vi "Read Config InI.vi"(0 "名称或相对路径":string="UserDefine.ini", 5 "error in (no error)":errorcluster caption="错误输入（无错误）") -> (14 "ParamSet":string[](array[string]), 15 "Other Params":string[](array[string]), 17 "In Stack":string[](array[string]), 18 "Out Stack":string[](array[string]), 19 "error out":errorcluster caption="错误输出")   [LabVIEW 2017]
uses:
  Global System.vi
  <vilib>/Utility/config.llb/NI_LVConfig.lvlib
panel:
  out "添加的路径":path
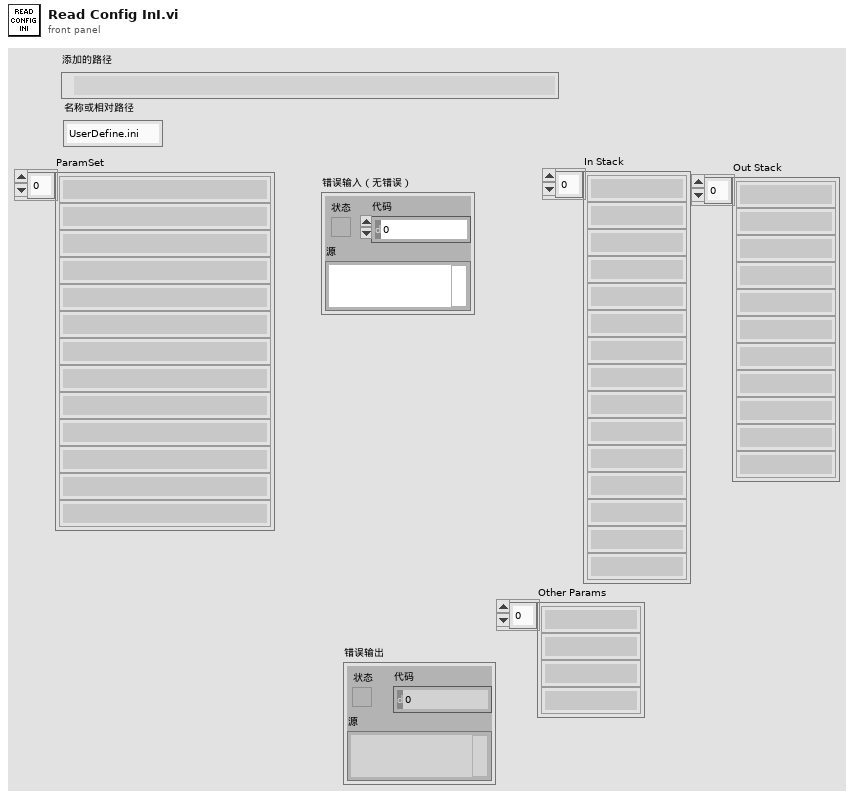
[diagram p1: front panel]
types:
  T1 = typedef "NI_LVConfig.lvlib/Config Data RefNum.ctl" = refnum<k1>
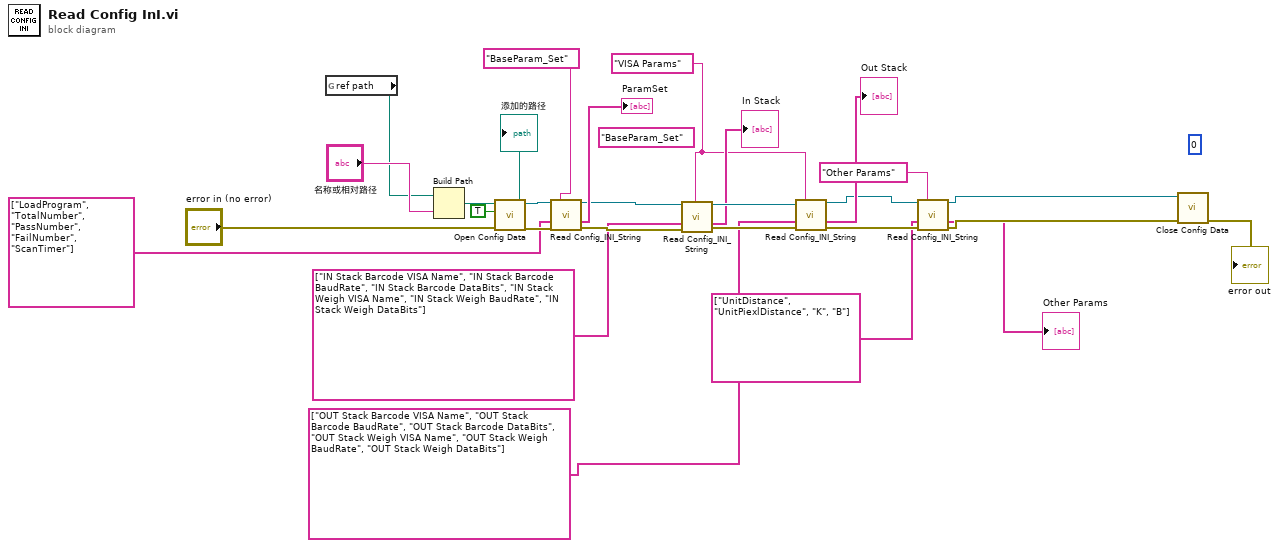
[diagram p0: block diagram]
diagram:
  w8 = "VISA Params" ("section")
  (unwired) "BaseParam_Set" ("section")
  (unwired) 0 ("索引")
  n1 = global read "Global System.vi" "ref path"() -> (w21:path)
  n2 = Build Path(base path=w21, name or relative path="名称或相对路径") -> (appended path=w24:path)
  "添加的路径" <- w24
  n3 = call <vilib>:"Open Config Data.vi"("error in (no error)"="error in (no error)", "create file if necessary (T)"=TRUE, "configuration file path"=w24) -> ("error out"=w26:errorcluster, "refnum"=w25:T1)  [unwired: 6 in, 1 out]
  n4 = call "Read Config_INI_String.vi"("refnum"=w25, "section"="BaseParam_Set", "Keys"=string[] ["LoadProgram", "TotalNumber", "PassNumber", "FailNumber", "ScanTimer"], "error in (no error)"=w26) -> ("refnum out"=w13:T1, "Outputs"=→"ParamSet":string[], "error out"=w16:errorcluster)  [unwired: 9 in]
  n5 = call "Read Config_INI_String.vi"("refnum"=w13, "section"=w8, "Keys"=string[] ["IN Stack Barcode VISA Name", "IN Stack Barcode BaudRate", "IN Stack Barcode DataBits", "IN Stack Weigh VISA Name", "IN Stack Weigh BaudRate", "IN Stack Weigh DataBits"], "error in (no error)"=w16) -> ("refnum out"=w15:T1, "Outputs"=→"In Stack":string[], "error out"=w14:errorcluster)  [unwired: 9 in]
  n6 = call "Read Config_INI_String.vi"("refnum"=w15, "section"=w8, "Keys"=string[] ["OUT Stack Barcode VISA Name", "OUT Stack Barcode BaudRate", "OUT Stack Barcode DataBits", "OUT Stack Weigh VISA Name", "OUT Stack Weigh BaudRate", "OUT Stack Weigh DataBits"], "error in (no error)"=w14) -> ("refnum out"=w7:T1, "Outputs"=→"Out Stack":string[], "error out"=w5:errorcluster)  [unwired: 9 in]
  n7 = call "Read Config_INI_String.vi"("refnum"=w7, "section"="Other Params", "Keys"=string[] ["UnitDistance", "UnitPiexlDistance", "K", "B"], "error in (no error)"=w5) -> ("refnum out"=w6:T1, "Outputs"=→"Other Params":string[], "error out"=w4:errorcluster)  [unwired: 9 in]
  n8 = call <vilib>:"Close Config Data.vi"("error in (no error)"=w4, "refnum"=w6) -> ("error out"=→"error out":errorcluster)  [unwired: 8 in, 1 out]
